vi "Version 1_Liquid Unit Detect.vi"(7 "Address (A)":string="A", 8 "error in":errorcluster, 11 "VISA Session In":refnum<visa-resource-name>="Alicat") -> (0 "error out":errorcluster, 1 "Liquid Unit?":enum32{"Gas", "Liquid"}(radio), 3 "VISA Session Out":refnum<visa-resource-name>)   [LabVIEW 2016]
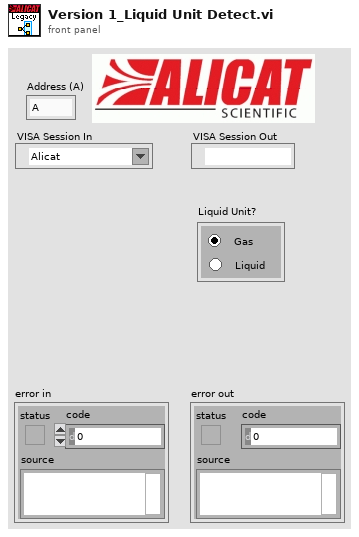
[diagram p1: front panel]
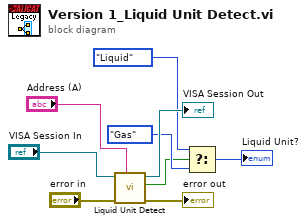
[diagram p0: block diagram]
diagram:
  n1 = call "Liquid Unit Detect.vi"("Unit ID (A)"="Address (A)", "error in"="error in", "VISA Session In"="VISA Session In") -> ("error out"=→"error out":errorcluster, "Liquid Device"=w1:bool, "VISA Session Out"=→"VISA Session Out":refnum<visa-resource-name>)  [unwired: 6 in]
  n2 = Select(t=enum32{"Gas", "Liquid"}."Liquid" ("Liquid Unit?"), s=w1, f=enum32{"Gas", "Liquid"}."Gas" ("Liquid Unit?")) -> (s? t:f=→"Liquid Unit?":enum32{"Gas", "Liquid"})
